vi "Control_Suction_Hi-Tec.vi"(0 "Suction rate (ml/min/ch)":dbl format="%.2f") -> (1 "Error Comments":string, 2 "Voltage Set":dbl format="%.2f")   [LabVIEW 2016]
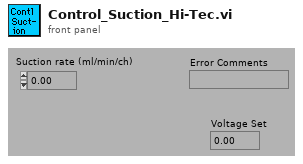
[diagram p1: front panel]
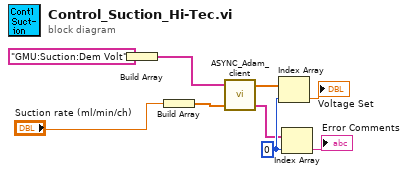
[diagram p0: block diagram]
diagram:
  w9 = 0 ("Index")
  n1 = Build Array("GMU:Suction:Dem Volt") -> (w5:string[])
  n2 = Build Array("Suction rate (ml/min/ch)") -> (w6:dbl[])
  n3 = call "ASYNC_Adam_client.vi"("Values"=w6, "Channel Names"=w5) -> ("Scan Comments"=w8:string[], "Calibrated Units"=w7:dbl[])  [unwired: 1 in]
  n4 = Index Array(array=w7, index=w9) -> (element=→"Voltage Set":dbl)
  n5 = Index Array(array=w8, index=w9) -> (element=→"Error Comments":string)
